vi "MecaDrivePoseEst2_SetVisionMeasurementStdDevs.vi"(9 "VisionMeasurementStdDevs":T1=[[0.9], [0.9], [0.9]], 11 "in MecaDrivePoseEstimate2":T2={"M_Vision_K"=[], "m_nominal_dT"=0.0, "m_PrevTime_Sec"=0.0, "Pose_Buffer"={"TimeStamps"=[], "DataArray"=[], "Min_TimeStamp"=0.0, "Max_TimeStamp"=0.0, "ItemCount"=0, "MaxBufferTime"=0.0}, "Meca_Drive_Odom"={"POSE"={"TRANSLATION"={"X"=0.0, "Y"=0.0}, "ROTATION"={"VALUE"=0.0, "COS"=1.0, "SIN"=0.0}}, "GyroOffset"={"VALUE"=0.0, "COS"=1.0, "SIN"=0.0}, "PreviousAngle"={"VALUE"=0.0, "COS"=1.0, "SIN"=0.0}, "Kinematics"={"FrontLeft"={"X"=0.0, "Y"=0.0}, "FrontRight"={"X"=0.0, "Y"=0.0}, "RearLeft"={"X"=0.0, "Y"=0.0}, "RearRight"={"X"=0.0, "Y"=0.0}, "InverseKinematics"=[[0.0, 1.0, -1.0, 0.0], [0.0, 1.0, 1.0, 0.0], [0.0, 1.0, 1.0, 0.0], [0.0, 1.0, -1.0, 0.0]], "ForwardKinematics"=[[0.0, 1.0, -1.0, 0.0], [0.0, 1.0, 1.0, 0.0], [0.0, 1.0, 1.0, 0.0], [0.0, 1.0, -1.0, 0.0]], "PrevCoR"={"X"=0.0, "Y"=0.0}}, "PreviousWheelPositions"={"FrontLeft"=0.0, "FrontRight"=0.0, "RearLeft"=0.0, "RearRight"=0.0, "P"=FALSE}}, "M_Q"=[[0.0], [0.0], [0.0]]} {"Meca_Drive_Odom"."PreviousWheelPositions"."RearRight" format="%19.3f"; "Meca_Drive_Odom"."PreviousWheelPositions"."RearLeft" format="%19.3f"; "Meca_Drive_Odom"."PreviousWheelPositions"."FrontRight" format="%19.3f"; "Meca_Drive_Odom"."PreviousWheelPositions"."FrontLeft" format="%19.3f"; "Meca_Drive_Odom"."Kinematics"."PrevCoR"."Y" format="%14.3f"; "Meca_Drive_Odom"."Kinematics"."PrevCoR"."X" format="%14.3f"; "Meca_Drive_Odom"."Kinematics"."RearRight"."Y" format="%14.3f"; "Meca_Drive_Odom"."Kinematics"."RearRight"."X" format="%14.3f"; "Meca_Drive_Odom"."Kinematics"."RearLeft"."Y" format="%14.3f"; "Meca_Drive_Odom"."Kinematics"."RearLeft"."X" format="%14.3f"; "Meca_Drive_Odom"."Kinematics"."FrontRight"."Y" format="%14.3f"; "Meca_Drive_Odom"."Kinematics"."FrontRight"."X" format="%14.3f"; "Meca_Drive_Odom"."Kinematics"."FrontLeft"."Y" format="%14.3f"; "Meca_Drive_Odom"."Kinematics"."FrontLeft"."X" format="%14.3f"; "Meca_Drive_Odom"."PreviousAngle"."SIN" format="%13.4f"; "Meca_Drive_Odom"."PreviousAngle"."COS" format="%13.4f"; "Meca_Drive_Odom"."PreviousAngle"."VALUE" format="%13.4f"; "Meca_Drive_Odom"."GyroOffset"."SIN" format="%13.4f"; "Meca_Drive_Odom"."GyroOffset"."COS" format="%13.4f"; "Meca_Drive_Odom"."GyroOffset"."VALUE" format="%13.4f"; "Meca_Drive_Odom"."POSE"."ROTATION"."SIN" format="%13.4f"; "Meca_Drive_Odom"."POSE"."ROTATION"."COS" format="%13.4f"; "Meca_Drive_Odom"."POSE"."ROTATION"."VALUE" format="%13.4f"; "Meca_Drive_Odom"."POSE"."TRANSLATION"."Y" format="%14.3f"; "Meca_Drive_Odom"."POSE"."TRANSLATION"."X" format="%14.3f"}) -> (0 "Size Coerced":bool, 3 "Out MecaDrivePoseEstimate2":T2={"M_Vision_K"=[], "m_nominal_dT"=0.0, "m_PrevTime_Sec"=0.0, "Pose_Buffer"={"TimeStamps"=[], "DataArray"=[], "Min_TimeStamp"=0.0, "Max_TimeStamp"=0.0, "ItemCount"=0, "MaxBufferTime"=0.0}, "Meca_Drive_Odom"={"POSE"={"TRANSLATION"={"X"=0.0, "Y"=0.0}, "ROTATION"={"VALUE"=0.0, "COS"=1.0, "SIN"=0.0}}, "GyroOffset"={"VALUE"=0.0, "COS"=1.0, "SIN"=0.0}, "PreviousAngle"={"VALUE"=0.0, "COS"=1.0, "SIN"=0.0}, "Kinematics"={"FrontLeft"={"X"=0.0, "Y"=0.0}, "FrontRight"={"X"=0.0, "Y"=0.0}, "RearLeft"={"X"=0.0, "Y"=0.0}, "RearRight"={"X"=0.0, "Y"=0.0}, "InverseKinematics"=[[0.0, 1.0, -1.0, 0.0], [0.0, 1.0, 1.0, 0.0], [0.0, 1.0, 1.0, 0.0], [0.0, 1.0, -1.0, 0.0]], "ForwardKinematics"=[[0.0, 1.0, -1.0, 0.0], [0.0, 1.0, 1.0, 0.0], [0.0, 1.0, 1.0, 0.0], [0.0, 1.0, -1.0, 0.0]], "PrevCoR"={"X"=0.0, "Y"=0.0}}, "PreviousWheelPositions"={"FrontLeft"=0.0, "FrontRight"=0.0, "RearLeft"=0.0, "RearRight"=0.0, "P"=FALSE}}, "M_Q"=[[0.0], [0.0], [0.0]]} {"Meca_Drive_Odom"."PreviousWheelPositions"."RearRight" format="%19.3f"; "Meca_Drive_Odom"."PreviousWheelPositions"."RearLeft" format="%19.3f"; "Meca_Drive_Odom"."PreviousWheelPositions"."FrontRight" format="%19.3f"; "Meca_Drive_Odom"."PreviousWheelPositions"."FrontLeft" format="%19.3f"; "Meca_Drive_Odom"."Kinematics"."PrevCoR"."Y" format="%14.3f"; "Meca_Drive_Odom"."Kinematics"."PrevCoR"."X" format="%14.3f"; "Meca_Drive_Odom"."Kinematics"."RearRight"."Y" format="%14.3f"; "Meca_Drive_Odom"."Kinematics"."RearRight"."X" format="%14.3f"; "Meca_Drive_Odom"."Kinematics"."RearLeft"."Y" format="%14.3f"; "Meca_Drive_Odom"."Kinematics"."RearLeft"."X" format="%14.3f"; "Meca_Drive_Odom"."Kinematics"."FrontRight"."Y" format="%14.3f"; "Meca_Drive_Odom"."Kinematics"."FrontRight"."X" format="%14.3f"; "Meca_Drive_Odom"."Kinematics"."FrontLeft"."Y" format="%14.3f"; "Meca_Drive_Odom"."Kinematics"."FrontLeft"."X" format="%14.3f"; "Meca_Drive_Odom"."PreviousAngle"."SIN" format="%13.4f"; "Meca_Drive_Odom"."PreviousAngle"."COS" format="%13.4f"; "Meca_Drive_Odom"."PreviousAngle"."VALUE" format="%13.4f"; "Meca_Drive_Odom"."GyroOffset"."SIN" format="%13.4f"; "Meca_Drive_Odom"."GyroOffset"."COS" format="%13.4f"; "Meca_Drive_Odom"."GyroOffset"."VALUE" format="%13.4f"; "Meca_Drive_Odom"."POSE"."ROTATION"."SIN" format="%13.4f"; "Meca_Drive_Odom"."POSE"."ROTATION"."COS" format="%13.4f"; "Meca_Drive_Odom"."POSE"."ROTATION"."VALUE" format="%13.4f"; "Meca_Drive_Odom"."POSE"."TRANSLATION"."Y" format="%14.3f"; "Meca_Drive_Odom"."POSE"."TRANSLATION"."X" format="%14.3f"})   [LabVIEW 2019, in "Trajectory_Library.lvlib"]
doc: "Sets the pose estimator's trust of global measurements. This might be used to change trust in vision measurements after the autonomous period, or to change trust as distance to a vision target increases.\n \nInputs:\n - inSwerveDrvPoseEst2 -- SwerveDrvPoseEst2 -- Data cluster\n - VisionMeasurementStdDevs -- <3,1> Matrix -- Standard deviations of the vision measurements. Increase these numbers to trust global measurements from vision less. This matrix is in the form [x, y, theta]Time, with units in meters and radians.\n\nOutputs:\n - outSwerveDrvPoseEst2 -- SwerveDrvPoseEst2 -- Updated data cluster\n - sizeCooerced -- boolean -- If TRUE, then the size of the vision measurement standard deviations was not 3,1. The size was modified to allow this routine to complete."
uses:
  Trajectory_Library.lvlib
  TypeDef/MECA_DRIVE_POSE_EST2.ctl
  <vilib>/Analysis/Matrix/Datatypes/RealMatrix.ctl
  TypeDef/TIME_INTERPOLATABLE_VARIANT.ctl
  TypeDef/MECA_DRIVE_ODOMETRY.ctl
  TypeDef/POSE2D.ctl
  TypeDef/TRANSLATION2D.ctl
  TypeDef/ROTATION2D.ctl
  TypeDef/MECA_DRIVE_KINEMATICS.ctl
  TypeDef/MECA_WHEEL_POSITIONS.ctl
  MatBuilder_Create.vi
  <vilib>/Analysis/Matrix/NI_Matrix.lvlib
panel:
  # "<3, 1>"
  # "<3, 1>"
  # "<3, 3>"
  # "<3, 1>"
  # "<3, 3>"
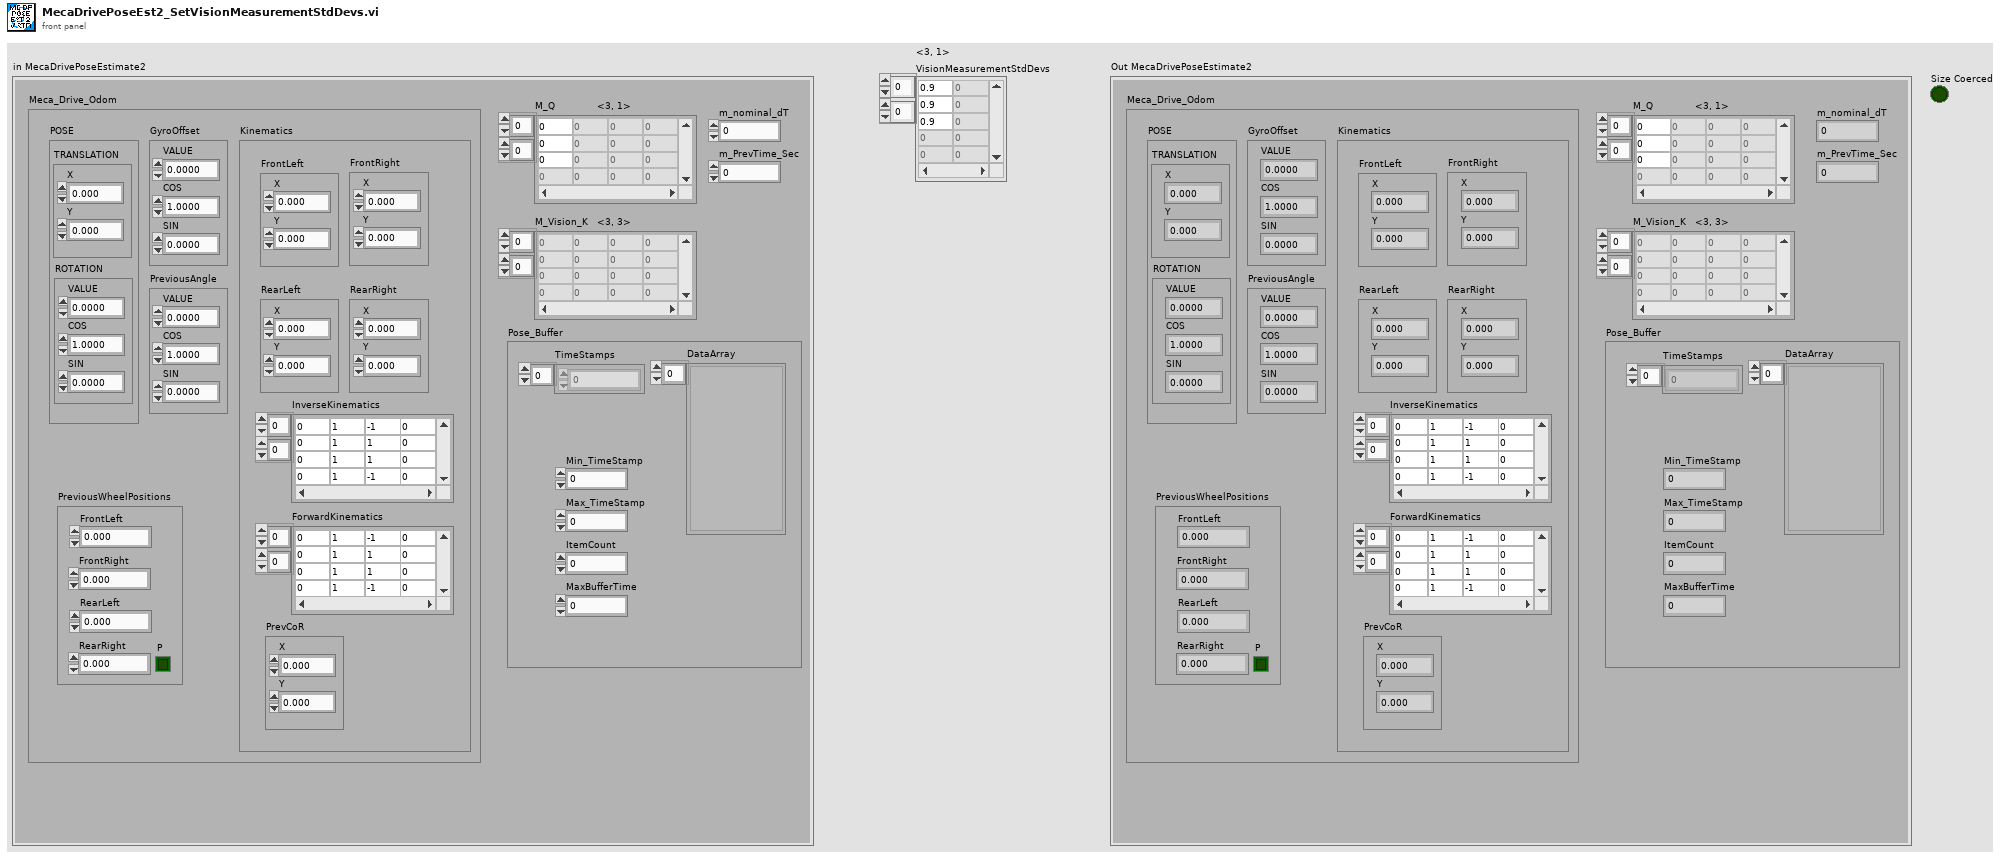
[diagram p1: front panel]
types:
  T1 = typedef "NI_Matrix.lvlib/RealMatrix.ctl" = dbl[][]
  T2 = typedef "Trajectory_Library.lvlib/MECA_DRIVE_POSE_EST2.ctl" = cluster{"M_Vision_K":T1, "m_nominal_dT":dbl, "m_PrevTime_Sec":dbl, "Pose_Buffer":T3, "Meca_Drive_Odom":T4, "M_Q":T1}
  T3 = typedef "Trajectory_Library.lvlib/TIME_INTERPOLATABLE_VARIANT.ctl" = cluster{"TimeStamps":dbl[], "DataArray":variant[], "Min_TimeStamp":dbl, "Max_TimeStamp":dbl, "ItemCount":i32, "MaxBufferTime":dbl}
  T4 = typedef "Trajectory_Library.lvlib/MECA_DRIVE_ODOMETRY.ctl" = cluster{"POSE":T5, "GyroOffset":T7, "PreviousAngle":T7, "Kinematics":T8, "PreviousWheelPositions":T9}
  T5 = typedef "Trajectory_Library.lvlib/POSE2D.ctl" = cluster{"TRANSLATION":T6, "ROTATION":T7}
  T6 = typedef "Trajectory_Library.lvlib/TRANSLATION2D.ctl" = cluster{"X":dbl, "Y":dbl}
  T7 = typedef "Trajectory_Library.lvlib/ROTATION2D.ctl" = cluster{"VALUE":dbl, "COS":dbl, "SIN":dbl}
  T8 = typedef "Trajectory_Library.lvlib/MECA_DRIVE_KINEMATICS.ctl" = cluster{"FrontLeft":T6, "FrontRight":T6, "RearLeft":T6, "RearRight":T6, "InverseKinematics":T1, "ForwardKinematics":T1, "PrevCoR":T6}
  T9 = typedef "Trajectory_Library.lvlib/MECA_WHEEL_POSITIONS.ctl" = cluster{"FrontLeft":dbl, "FrontRight":dbl, "RearLeft":dbl, "RearRight":dbl, "P":bool}
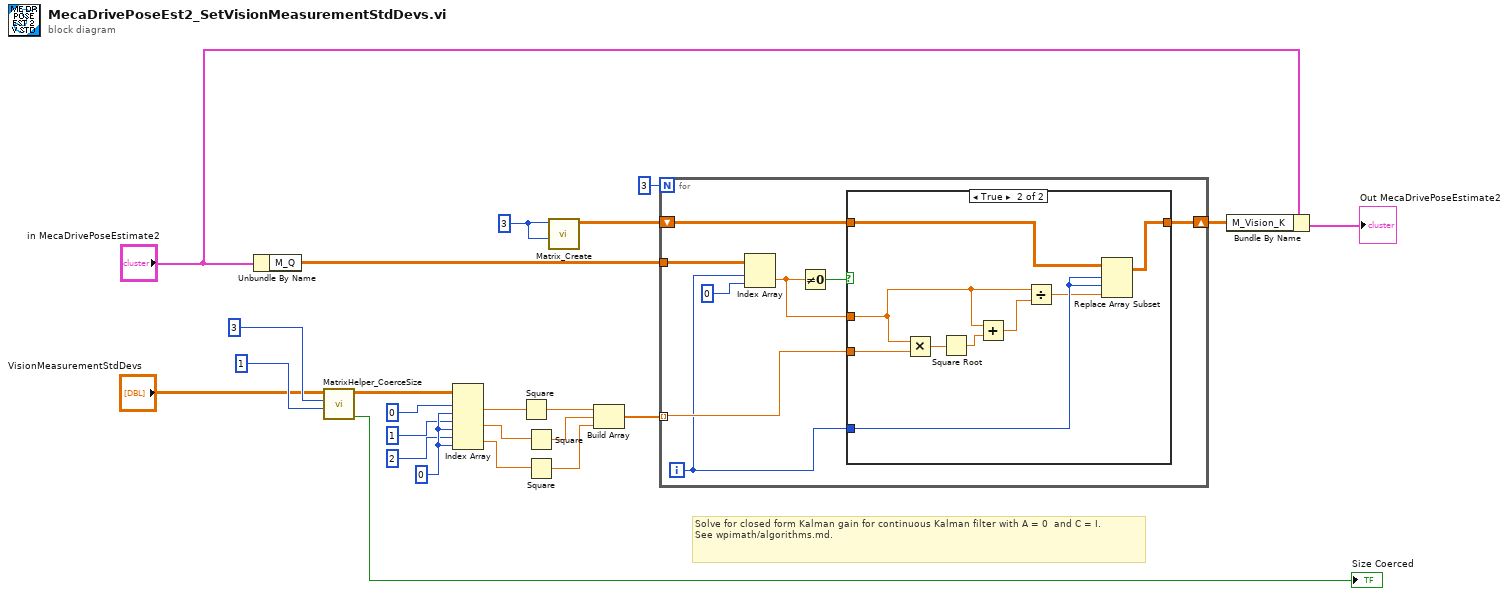
[diagram p0: block diagram]
diagram:
  w5 = 3 ("Rows")
  w17 = 0 ("index (col)")
  # "Solve for closed form Kalman gain for continuous Kalman filter with A = 0  and C = I. \nSee wpimath/algorithms.md."
  n1 = Unbundle By Name("in MecaDrivePoseEstimate2") -> ("M_Q"=w2:T1)
  n2 = call "MatrixHelper_CoerceSize.vi"("Columns"=1 ("Outputs"), "Rows"=3 ("States"), "input matrix"="VisionMeasurementStdDevs") -> ("Coerced"=→"Size Coerced":bool, "output matrix"=w6:T1)  [unwired: 7 in]
  n3 = Index Array(array=w6, index (row) #1=0 ("index (row)"), index (col) #1=w17, index (row) #2=1 ("index (row)"), index (col) #2=w17, index (row) #3=2 ("index (row)"), index (col) #3=w17) -> (element #1=w14:dbl, element #2=w13:dbl, element #3=w12:dbl)
  n4 = Square(x=w14) -> (x^2=w11:dbl)
  n5 = Square(x=w13) -> (x^2=w10:dbl)
  n6 = Square(x=w12) -> (x^2=w9:dbl)
  n7 = call "Matrix_Create.vi"("Columns"=w5, "Rows"=w5) -> ("output matrix"=w4:T1)  [unwired: 9 in]
  n8 = Build Array(w11, w10, w9) -> (w7:dbl[])
  n9 = for {
    N: 3 -> [_]
    tunnel: w7 -> [w25] mode=indexing
    tunnel: w2 -> [w30]
    shift-right: [w27] -> w1
    shift-left: w4 -> [w28]
    i -> [w24]
    n10 = Index Array(array=w30, index (row)=w24, index (col)=0) -> (element=w26:dbl)
    n11 = Not Equal To 0?(x=w26) -> (x != 0?=w29:bool)
    n12 = case shown="True" w29 {
      tunnel: w28 -> [w32 w36]
      tunnel: [w32 w35] -> w27
      tunnel: w26 -> [_ w38]
      tunnel: w25 -> [_ w41]
      tunnel: w24 -> [_ w34]
      frame False {
      }
      frame True {
        n13 = Multiply(x=w38, y=w41) -> (x*y=w40:dbl)
        n14 = Square Root(x=w40) -> (sqrt(x)=w39:dbl)
        n15 = Add(x=w38, y=w39) -> (x+y=w37:dbl)
        n16 = Divide(x=w38, y=w37) -> (x/y=w33:dbl)
        n17 = Replace Array Subset(array=w36, new element=w33, index (row)=w34, index (col)=w34) -> (w35:T1)
      }
    }
  }
  n18 = Bundle By Name(cluster="in MecaDrivePoseEstimate2", "M_Vision_K"=w1) -> (→"Out MecaDrivePoseEstimate2":T2)
